vi "Number of Address Map Elements.vi"(2 "niUSRP Tx DSP v2 FPGA":refnum<class "niUSRP Tx DSP v2 FPGA.lvclass">) -> (6 "number of elements":u8)   [LabVIEW 2025, in "niUSRP Tx DSP v2 FPGA.lvclass"]
uses:
  niUSRP Tx DSP v2 FPGA.lvclass
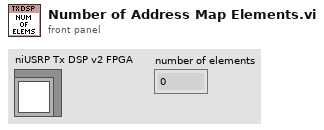
[diagram p1: front panel]
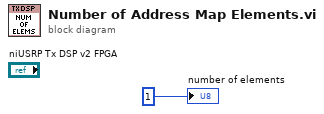
[diagram p0: block diagram]
diagram:
  "number of elements" <- u8 1 ("number of elements")
